vi "Initialize.vi"(4 "id":string, 8 "error in (no error)":errorcluster, 9 "Style":string, 10 "Dot":T1, 11 "Dot in":refnum<class "Dot.lvclass">) -> (0 "error out":errorcluster, 3 "Dot out":refnum<class "Dot.lvclass">)   [LabVIEW 2019, in "Dot.lvclass"]
uses:
  Dot.lvclass
  CircleData.ctl
  CSSProperties/CSSProperties.lvclass
  Dot.lvclass/Dot.ctl
  Write Style.vi
  Write cx.vi
  Write cy.vi
  Write r.vi
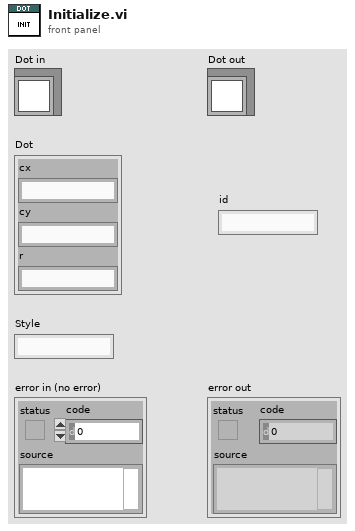
[diagram p1: front panel]
types:
  T1 = typedef "Dot.lvclass/CircleData.ctl" = cluster{"cx":string, "cy":string, "r":string}
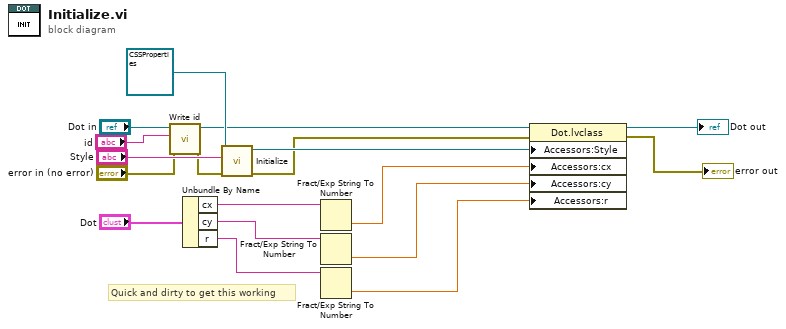
[diagram p0: block diagram]
diagram:
  # "Quick and dirty to get this working"
  n1 = call-dynamic "Write id.vi"("error in (no error)"="error in (no error)", "id"="id", "SVG Object in"="Dot in") -> ("error out"=w2:errorcluster, "SVG Object out"=w4:refnum<class "Dot.lvclass">)  [unwired: 7 in]
  n2 = Unbundle By Name("Dot") -> ("cx"=w11:string, "cy"=w8:string, "r"=w7:string)
  n3 = call "Initialize.vi"("error in (no error)"=w2, "Properties String"="Style", "CSSProperties in"=refnum<class "CSSProperties.lvclass"> refnum) -> ("error out"=w13:errorcluster, "CSSProperties out"=w14:refnum<class "CSSProperties.lvclass">)  [unwired: 7 in]
  n4 = Fract/Exp String To Number(string=w11) -> (number=w10:dbl)  [unwired: 3 in, 1 out]
  n5 = Fract/Exp String To Number(string=w8) -> (number=w9:dbl)  [unwired: 3 in, 1 out]
  n6 = Fract/Exp String To Number(string=w7) -> (number=w6:dbl)  [unwired: 3 in, 1 out]
  n7 = property class="Dot.lvclass"(reference=w4, error in=w13, "Accessors:Style"=w14, "Accessors:cx"=w10, "Accessors:cy"=w9, "Accessors:r"=w6) -> (reference out=→"Dot out":refnum<class "Dot.lvclass">, error out=→"error out":errorcluster)
